vi "Add Header.vi"(8 "error in (no error)":errorcluster, 11 "CSV File Sink in":refnum<class "CSV File Sink.lvclass">) -> (0 "error out":errorcluster, 3 "CSV File Sink out":refnum<class "CSV File Sink.lvclass">)   [LabVIEW 2016, in "Stream Log.lvlib" / "CSV File Sink.lvclass"]
doc: "--\nCopyright © 2017 Composed SystemsI All rights reserved.\n\nAuthor: Jon McBee <jon.mcbee@composed.io>\n\nThis library is provided \"AS IS\" ,WITHOUT WARRANTIES OR\nCONDITIONS OF ANY KIND, either express or implied.\n\nComposed Systems -- composed.io\n\nStream 0.0.1.1\nJon McBee - Composed Systems\nCopyright (c) 2017, Composed Systems"
uses:
  <userlib>/Composed Systems/Stream/Log/CSV File Sink/CSV File Sink.lvclass
  C:/Program Files (x86)/National Instruments/LabVIEW 2016/user.lib/Composed Systems/Stream/Log/Text File Sink/Text File Sink.lvclass
  <userlib>/Composed Systems/Stream/Log/CSV File Sink/CSV File Sink.lvclass/CSV File Sink.ctl
  <userlib>/Composed Systems/Stream/Log/Text File Sink/Text File Sink.lvclass/Text File Sink.ctl
  <userlib>/Composed Systems/Stream/Log/Text File Sink/Text File Sink.lvclass
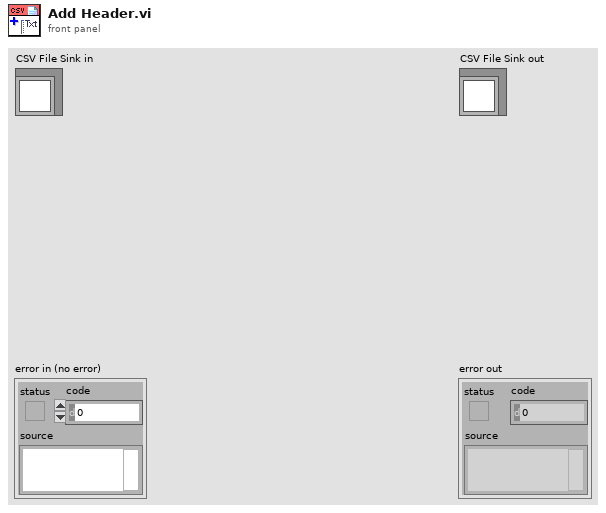
[diagram p1: front panel]
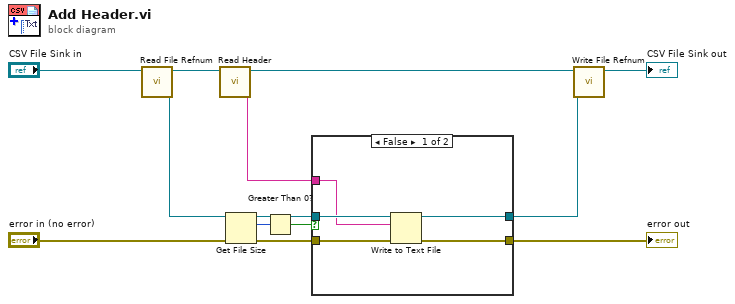
[diagram p0: block diagram]
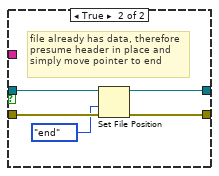
[diagram p2: hidden frame]
diagram:
  n1 = call <userlib>:"Read File Refnum.vi"("Text File Sink in"="CSV File Sink in") -> ("File Refnum"=w2:refnum<file>, "Text File Sink out"=w11:refnum<class "CSV File Sink.lvclass">)  [unwired: 9 in]
  n2 = call <userlib>:"Read Header.vi"("CSV File Sink in"=w11) -> ("Header"=w3:string, "CSV File Sink out"=w10:refnum<class "CSV File Sink.lvclass">)  [unwired: 9 in]
  n3 = Get File Size(file=w2, error in="error in (no error)") -> (refnum out=w6:refnum<file>, size (in bytes)=w9:i64, 0:w8:errorcluster)
  n4 = Greater Than 0?(x=w9) -> (x > 0?=w7:bool)
  n5 = case shown="False" w7 {
    tunnel: w8 -> [w18 w23]
    tunnel: w6 -> [w17 w22]
    tunnel: [w14 w20] -> w4
    tunnel: [w15 w19] -> w1
    tunnel: w3 -> [w16 _]
    frame False {
      n6 = Write to Text File(file (use dialog)=w17, text=w16, error in=w18) -> (refnum out=w15:refnum<file>, error out=w14:errorcluster)  [unwired: 2 out]
    }
    frame True {
      # "file already has data, therefore\npresume header in place and\nsimply move pointer to end"
      n7 = Set File Position(refnum=w22, from (0:start)=enum16{"start", "end", "current"}."end", error in=w23) -> (refnum out=w19:refnum<file>, error out=w20:errorcluster)  [unwired: 1 out]
    }
  }
  "error out" <- w4
  n8 = call <userlib>:"Write File Refnum.vi"("File Refnum"=w1, "Text File Sink in"=w10) -> ("Text File Sink out"=→"CSV File Sink out":refnum<class "CSV File Sink.lvclass">)  [unwired: 9 in]
